vi "reset port-odor ring StringsAndValues[] (sub-vi).vi"(8 "error in (no error)":errorcluster, 11 "port-odor ring refnum":refnum<vi>) -> (0 "error out":errorcluster, 3 "port-odor ring refnum out":refnum<vi>)   [LabVIEW 2021]
uses:
  type-defs/port-odor ring (type def).ctl
panel:
  in  "port-odor ring (reference)":T1 items=["off"]
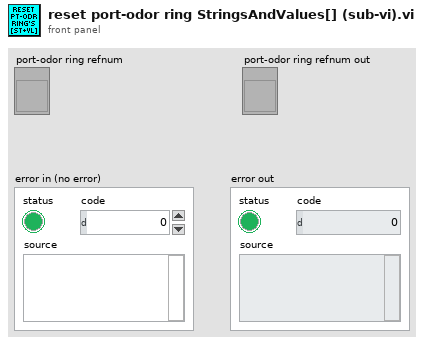
[diagram p1: front panel]
types:
  T1 = typedef "port-odor ring (type def).ctl" = u16
  T2 = typedef "LVStringsAndValuesArrayTypeDef_U16.ctl" = cluster{"String":string, "Value":u16}[]
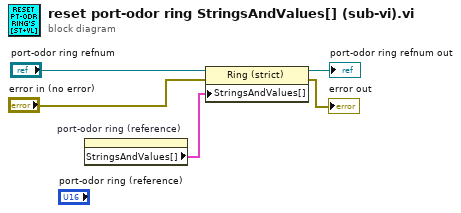
[diagram p0: block diagram]
diagram:
  n1 = property on="port-odor ring (reference)" class="Ring (strict)"() -> ("StringsAndValues[]"=w4:T2)  [unwired: 2 in, 2 out]
  n2 = property class="Ring (strict)"(reference="port-odor ring refnum", error in="error in (no error)", "StringsAndValues[]"=w4) -> (reference out=→"port-odor ring refnum out":refnum<vi>, error out=→"error out":errorcluster)
